vi "Aero_tunnel_monitor2.vi"() -> ()   [LabVIEW 2010]
uses:
  Aero_Tunnel_Server_Global.vi
panel:
  out "Road Info":string
  in  "stop":bool
  out "Lift":dbl caption="N" format="%#.2f"
  out "Pitch":dbl caption="N.m" format="%#.2f"
  out "Drag":dbl caption="N" format="%#.2f"
  out "Side-Force":dbl caption="N" format="%#.2f"
  out "Yaw":dbl caption="N.m" format="%#.2f"
  out "Roll":dbl caption="N.m" format="%#.2f"
  out "SmAD Data":dbl[](array[numeric]) format="%.2f"
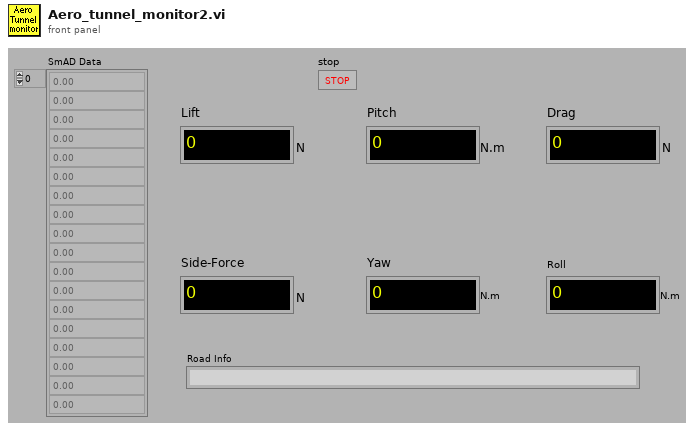
[diagram p1: front panel]
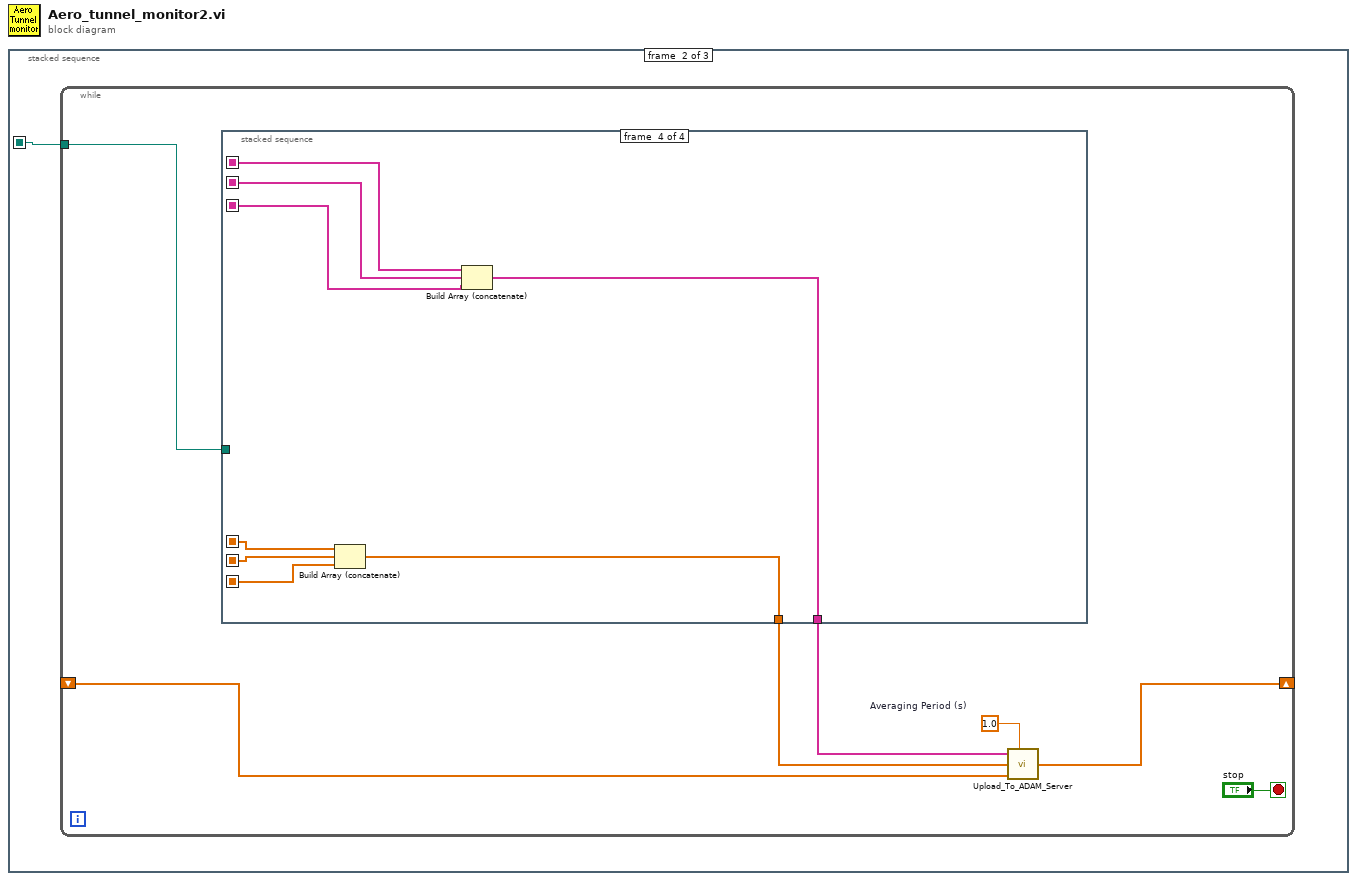
[diagram p0: block diagram]
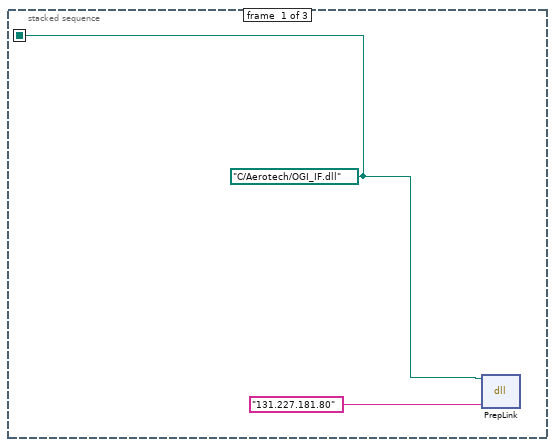
[diagram p2: hidden frame]
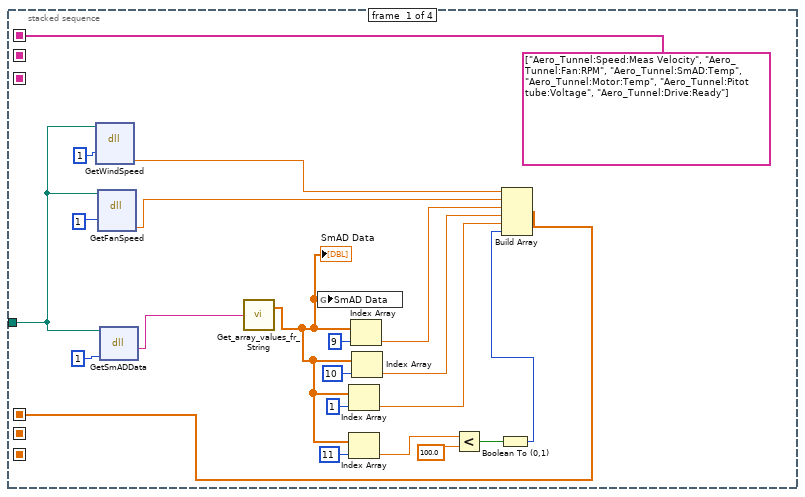
[diagram p3: hidden frame]
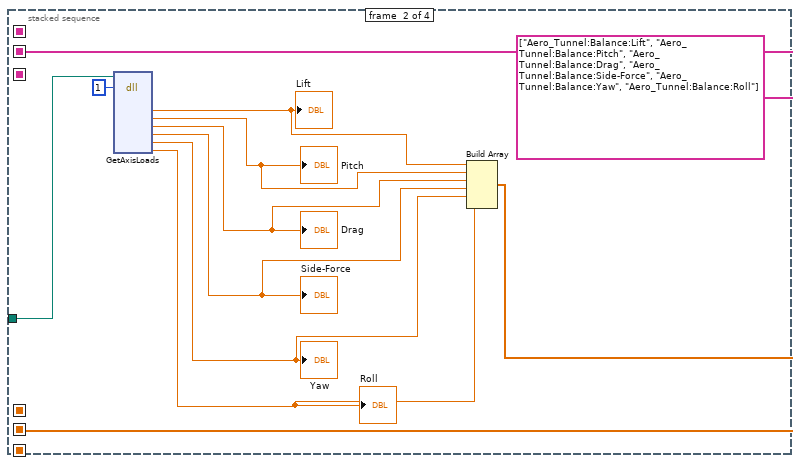
[diagram p4: hidden frame]
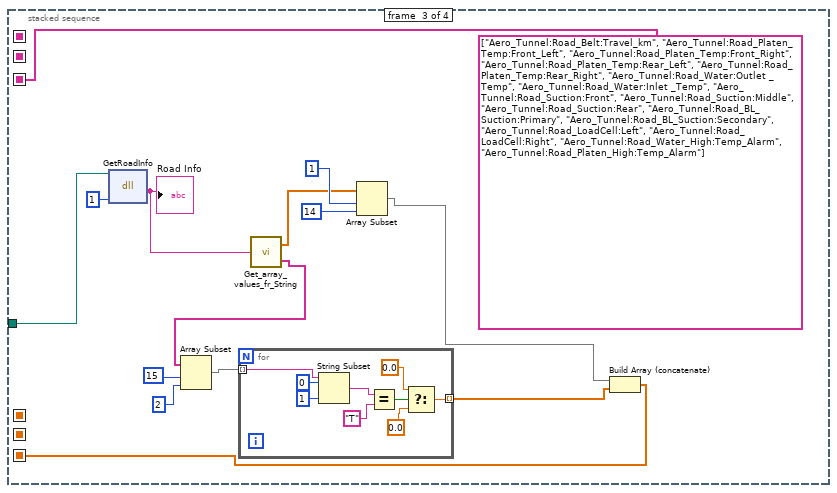
[diagram p5: hidden frame]
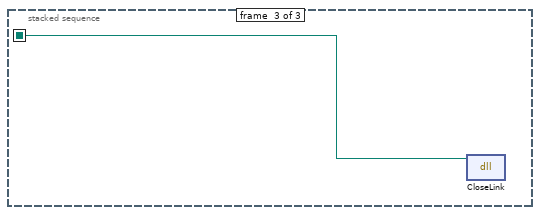
[diagram p6: hidden frame]
diagram:
  n1 = stacked-sequence {
    seq-local: [w1 _ _] -> [_ w3 w73]
    frame #0 {
      w1 = path "C:/Aerotech/OGI_IF.dll" ("path in")
      n2 = dll-call lib="C:/Aerotech/Drivers/OGI_IF.dll" fn="PrepLink"(path in=w1, "IPAddress"="131.227.181.80") -> ()  [unwired: 2 in, 4 out]
    }
    frame #1 {
      n3 = while {
        shift-right: [w10] -> _
        shift-left: _ -> [w8]
        tunnel: w3 -> [w5]
        stop <- "stop" stop-if-true
        w6 = 1.0  # Averaging Period (s)
        n4 = stacked-sequence {
          seq-local: [string[] ["Aero_Tunnel:Speed:Meas Velocity", "Aero_Tunnel:Fan:RPM", "Aero_Tunnel:SmAD:Temp", "Aero_Tunnel:Motor:Temp", "Aero_Tunnel:Pitot tube:Voltage", "Aero_Tunnel:Drive:Ready"] ("Channel Names") _ _ _] -> [_ _ _ w72]
          seq-local: [w19 _ _ _] -> [_ _ _ w70]
          seq-local: [_ string[] ["Aero_Tunnel:Balance:Lift", "Aero_Tunnel:Balance:Pitch", "Aero_Tunnel:Balance:Drag", "Aero_Tunnel:Balance:Side-Force", "Aero_Tunnel:Balance:Yaw", "Aero_Tunnel:Balance:Roll"] ("Channel Names") _ _] -> [_ _ _ w71]
          seq-local: [_ w40 _ _] -> [_ _ _ w69]
          seq-local: [_ _ w43 _] -> [_ _ _ w65]
          seq-local: [_ _ string[] ["Aero_Tunnel:Road_Belt:Travel_km", "Aero_Tunnel:Road_Platen_Temp:Front_Left", "Aero_Tunnel:Road_Platen_Temp:Front_Right", "Aero_Tunnel:Road_Platen_Temp:Rear_Left", "Aero_Tunnel:Road_Platen_Temp:Rear_Right", "Aero_Tunnel:Road_Water:Outlet _Temp", "Aero_Tunnel:Road_Water:Inlet _Temp", "Aero_Tunnel:Road_Suction:Front", "Aero_Tunnel:Road_Suction:Middle", "Aero_Tunnel:Road_Suction:Rear", "Aero_Tunnel:Road_BL_Suction:Primary", "Aero_Tunnel:Road_BL_Suction:Secondary", "Aero_Tunnel:Road_LoadCell:Left", "Aero_Tunnel:Road_LoadCell:Right", "Aero_Tunnel:Road_Water_High:Temp_Alarm", "Aero_Tunnel:Road_Platen_High:Temp_Alarm"] ("Channel Names") _] -> [_ _ _ w66]
          tunnel: [_ _ _ w68] -> w9
          tunnel: [_ _ _ w67] -> w7
          tunnel: w5 -> [w11 w38 w54 _]
          frame #0 {
            n5 = dll-call lib="C:/Aerotech/Drivers/OGI_IF.dll" fn="GetWindSpeed"(path in=w11, "Enable"=1) -> ("Windspeed_M/s"=w12:dbl)  [unwired: 3 in, 4 out]
            n6 = dll-call lib="C:/Aerotech/Drivers/OGI_IF.dll" fn="GetFanSpeed"(path in=w11, "Enable"=1) -> ("FanSpeedinRPM"=w13:dbl)  [unwired: 3 in, 4 out]
            n7 = dll-call lib="C:/Aerotech/Drivers/OGI_IF.dll" fn="GetSmADData"(path in=w11, "Enable"=1) -> ("SmAD Data String"=w16:string)  [unwired: 2 in, 3 out]
            n8 = call "Get_array_values_fr_String.vi"("String Value"=w16) -> ("Numeric Array"=w24:dbl[])  [unwired: 1 out]
            "SmAD Data" <- w24
            n9 = global write "Aero_Tunnel_Server_Global.vi" "SmAD Data"(w24) -> ()
            n10 = Index Array(array=w24, index=1) -> (element=w26:dbl)
            n11 = Index Array(array=w24, index=11) -> (element=w23:dbl)
            n12 = Index Array(array=w24, index=9) -> (element=w29:dbl)
            n13 = Index Array(array=w24, index=10) -> (element=w28:dbl)
            n14 = Less?(x=w23, y=100.0) -> (x < y?=w21:bool)
            n15 = Boolean To (0,1)(Boolean=w21) -> (0, 1=w20:i16)
            n16 = Build Array(w12, w13, w29, w28, w26, w20) -> (w19:dbl[])
          }
          frame #1 {
            n17 = dll-call lib="C:/Aerotech/Drivers/OGI_IF.dll" fn="GetAxisLoads"(path in=w38, "Enable"=1) -> ("Lift"=w37:dbl, "Pitch"=w36:dbl, "Drag"=w35:dbl, "side"=w34:dbl, "Yaw"=w33:dbl, "Roll"=w32:dbl)  [unwired: 3 in, 9 out]
            "Lift" <- w37
            "Pitch" <- w36
            "Drag" <- w35
            "Side-Force" <- w34
            "Yaw" <- w33
            "Roll" <- w32
            n18 = Build Array(w37, w36, w35, w34, w33, w32) -> (w40:dbl[])
          }
          frame #2 {
            n19 = dll-call lib="C:/Aerotech/Drivers/OGI_IF.dll" fn="GetRoadInfo"(path in=w54, "Enable"=1) -> ("Road Info"=w53:string)  [unwired: 3 in, 2 out]
            "Road Info" <- w53
            n20 = call "Get_array_values_fr_String.vi"("String Value"=w53) -> ("Numeric Array"=w50:dbl[], "String array"=w48:string[])
            n21 = Array Subset(array=w48, index=15, length=2) -> (w46:string[])
            n22 = for {
              tunnel: w46 -> [w62] mode=indexing
              tunnel: [w56] -> w45 mode=indexing
              n23 = String Subset(string=w62, offset (0)=0, length (rest)=1 ("length (rest)")) -> (substring=w61:string)
              n24 = Equal?(x=w61, y="T") -> (x = y?=w59:bool)
              n25 = Select(t=0.0, s=w59, f=0.0) -> (s? t:f=w56:dbl)
            }
            n26 = Array Subset(array=w50, index=1, length=14) -> (w44:dbl[])
            n27 = Build Array (concatenate)(w44, w45) -> (w43:dbl[])
          }
          frame #3 {
            n28 = Build Array (concatenate)(w70, w69, w65) -> (w68:dbl[])
            n29 = Build Array (concatenate)(w72, w71, w66) -> (w67:string[])
          }
        }
        n30 = call "Upload_To_ADAM_Server.vi"("Channel Names"=w7, "Averaging Period (s)"=w6, "Channel Values"=w9, "Shift In"=w8) -> ("Shift Out"=w10:dbl[])  [unwired: 1 out]
      }
    }
    frame #2 {
      n31 = dll-call lib="C:/Aerotech/Drivers/OGI_IF.dll" fn="CloseLink"(path in=w73) -> ()  [unwired: 2 in, 3 out]
    }
  }
